vi "LED_Rainbow.vi"() -> (0 "B":dbl, 1 "G":dbl, 2 "R":dbl)   [LabVIEW 2018]
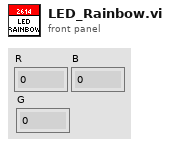
[diagram p1: front panel]
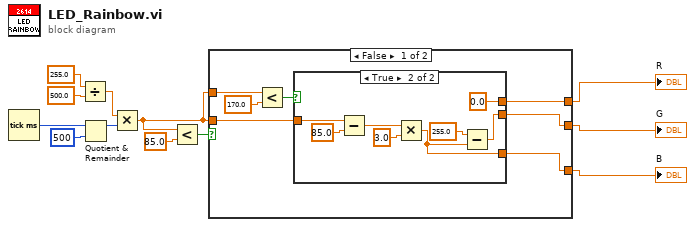
[diagram p0: block diagram]
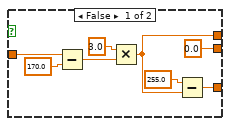
[diagram p2: hidden frame]
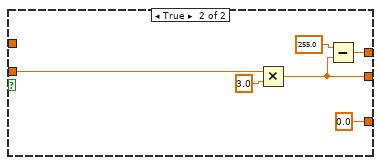
[diagram p3: hidden frame]
diagram:
  n1 = Tick Count (ms)() -> (millisecond timer value=w12:u32)
  n2 = Divide(x=255.0, y=500.0) -> (x/y=w9:dbl)
  n3 = Quotient & Remainder(x=w12, y=u32 500) -> (x-y*floor(x/y)=w10:u32)  [unwired: 1 out]
  n4 = Multiply(x=w9, y=w10) -> (x*y=w4:dbl)
  n5 = Less?(x=w4, y=85.0) -> (x < y?=w5:bool)
  n6 = case shown="False" w5 {
    tunnel: w4 -> [w16 w41]
    tunnel: [w15 w38] -> w3
    tunnel: [w14 0.0] -> w2
    tunnel: [w13 w36] -> w1
    tunnel: w4 -> [w18 _]
    frame False {
      n7 = Less?(x=w18, y=170.0) -> (x < y?=w19:bool)
      n8 = case shown="True" w19 {
        tunnel: w16 -> [w27 w35]
        tunnel: [w22 0.0] -> w15
        tunnel: [w21 w29] -> w14
        tunnel: [0.0 w28] -> w13
        frame False {
          n9 = Subtract(x=w27, y=170.0) -> (x-y=w24:dbl)
          n10 = Multiply(x=3.0, y=w24) -> (x*y=w22:dbl)
          n11 = Subtract(x=255.0, y=w22) -> (x-y=w21:dbl)
        }
        frame True {
          n12 = Subtract(x=w35, y=85.0) -> (x-y=w31:dbl)
          n13 = Multiply(x=w31, y=3.0) -> (x*y=w29:dbl)
          n14 = Subtract(x=255.0, y=w29) -> (x-y=w28:dbl)
        }
      }
    }
    frame True {
      n15 = Multiply(x=w41, y=3.0) -> (x*y=w36:dbl)
      n16 = Subtract(x=255.0, y=w36) -> (x-y=w38:dbl)
    }
  }
  "R" <- w3
  "G" <- w1
  "B" <- w2
